vi "set_all_ai_tc_types.vi"(8 "error in (no error)":errorcluster, 9 "Deafult AI type":string, 10 "All AI types":string[](array[string]), 11 "Modbus Master in":refnum<class "Modbus Master.lvclass">) -> (0 "error out":errorcluster, 3 "Modbus Master out":refnum<class "Modbus Master.lvclass">)   [LabVIEW 2018]
uses:
  <vilib>/NI/Modbus Library/API/Master/Modbus Master.lvclass
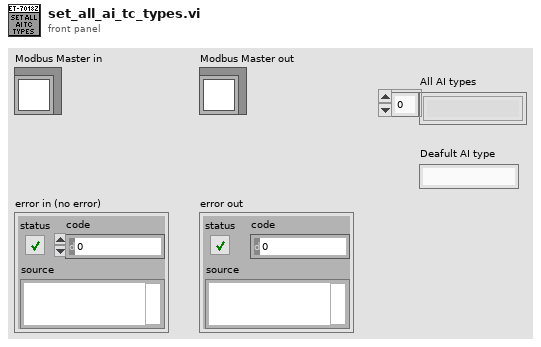
[diagram p1: front panel]
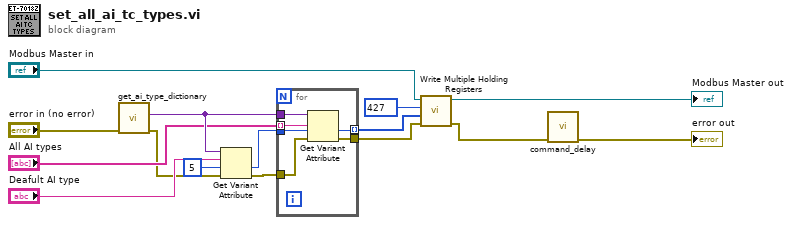
[diagram p0: block diagram]
diagram:
  n1 = call "get_ai_type_dictionary.vi"("error in (no error)"="error in (no error)") -> ("error out"=w5:errorcluster, "AI type dictionary"=w10:variant)  [unwired: 9 in]
  n2 = Get Variant Attribute(Variant=w10, name="Deafult AI type", default value (empty Variant)=5, error in=w5) -> (value=w8:i32, error out=w6:errorcluster)  [unwired: 2 out]
  n3 = for {
    tunnel: w10 -> [w21]
    tunnel: w8 -> [w20]
    tunnel: "All AI types" -> [w19] mode=indexing
    tunnel: [w18] -> w3 mode=indexing
    tunnel: w6 -> [w17]
    tunnel: [w16] -> w4
    n4 = Get Variant Attribute(Variant=w21, name=w19, default value (empty Variant)=w20, error in=w17) -> (value=w18:i32, error out=w16:errorcluster)  [unwired: 2 out]
  }
  n5 = call-dynamic "Write Multiple Holding Registers.vi"("error in"=w4, "registers to write"=w3, "starting address"=u16 427, "Modbus master in"="Modbus Master in") -> ("error out"=w2:errorcluster, "Modbus master out"=→"Modbus Master out":refnum<class "Modbus Master.lvclass">)  [unwired: 6 in]
  n6 = call "command_delay.vi"("error in (no error)"=w2) -> ("error out"=→"error out":errorcluster)  [unwired: 10 in]
